vi "WLAN_Scrambler.vi"(11 "input bit stream":i8[](array[numeric])) -> (2 "scrambled bits":i8[](array[numeric]), 3 "scrambler initial bit":i8[](array[numeric]))   [LabVIEW 2022 SP3]
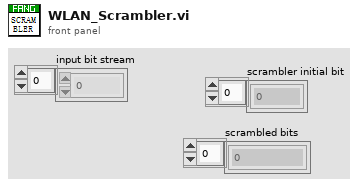
[diagram p1: front panel]
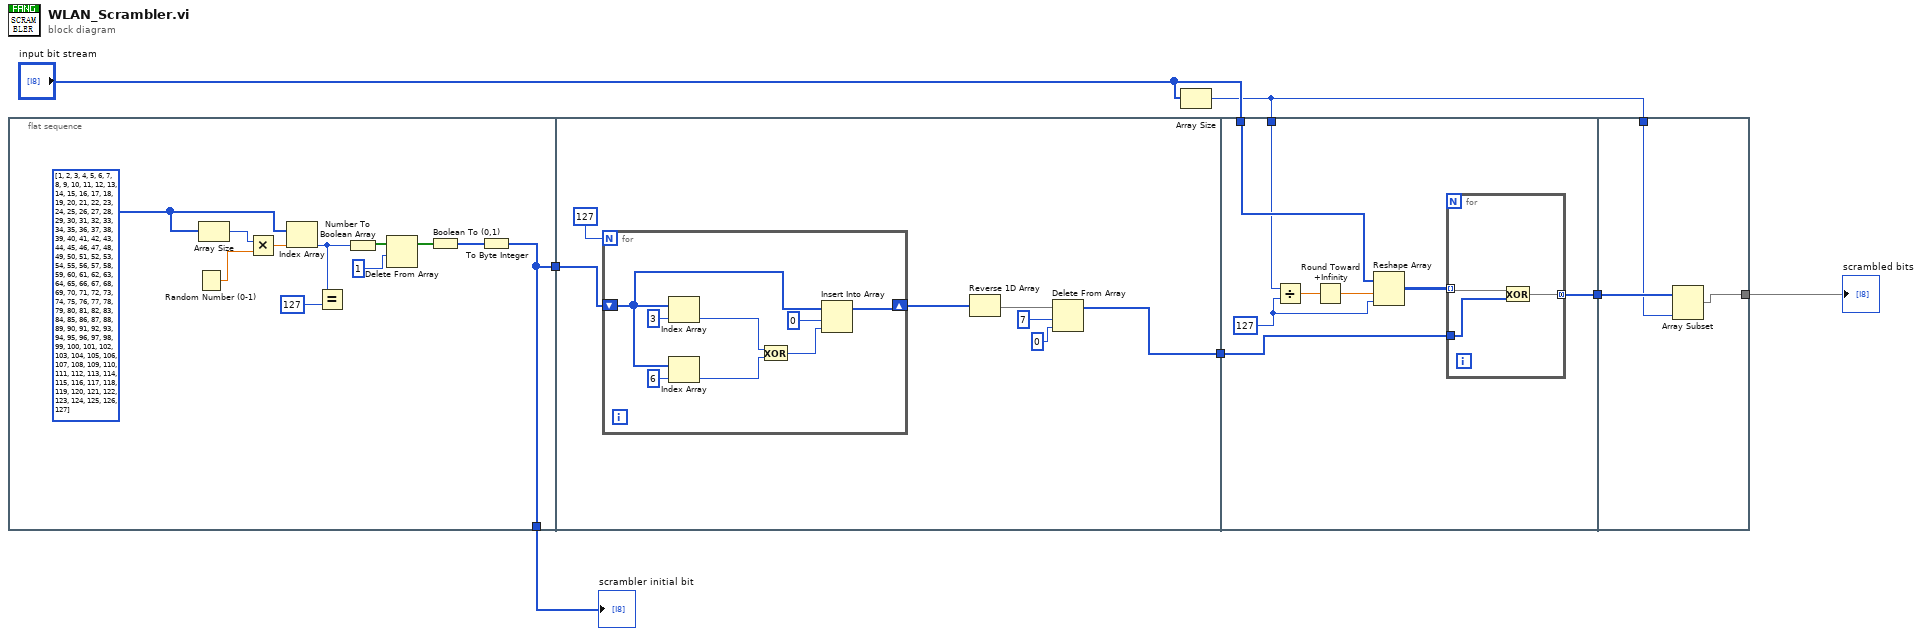
[diagram p0: block diagram]
diagram:
  n1 = flat-sequence {
    tunnel: [w8] -> w7
    tunnel: [w8] -> w6
    tunnel: w7 -> [w25]
    tunnel: [w19] -> w5
    tunnel: "input bit stream" -> [w40]
    tunnel: w5 -> [w36]
    tunnel: [w35] -> w3
    tunnel: w1 -> [w34]
    tunnel: [w45] -> w4
    tunnel: w3 -> [w47]
    tunnel: w1 -> [w46]
    frame #0 {
      w15 = i8[] [1, 2, 3, 4, 5, 6, 7, 8, 9, 10, 11, 12, 13, 14, 15, 16, 17, 18, 19, 20, 21, 22, 23, 24, 25, 26, 27, 28, 29, 30, 31, 32, 33, 34, 35, 36, 37, 38, 39, 40, 41, 42, 43, 44, 45, 46, 47, 48, 49, 50, 51, 52, 53, 54, 55, 56, 57, 58, 59, 60, 61, 62, 63, 64, 65, 66, 67, 68, 69, 70, 71, 72, 73, 74, 75, 76, 77, 78, 79, 80, 81, 82, 83, 84, 85, 86, 87, 88, 89, 90, 91, 92, 93, 94, 95, 96, 97, 98, 99, 100, 101, 102, 103, 104, 105, 106, 107, 108, 109, 110, 111, 112, 113, 114, 115, 116, 117, 118, 119, 120, 121, 122, 123, 124, 125, 126, 127] ("Array")
      n2 = Random Number (0-1)() -> (number: 0 to 1=w17:dbl)
      n3 = Array Size(array=w15) -> (size(s)=w18:i32)
      n4 = Multiply(x=w18, y=w17) -> (x*y=w16:dbl)
      n5 = Index Array(array=w15, index=w16) -> (element=w14:i8)
      n6 = Equal?(x=w14, y=i8 127) -> ()  [unwired: 1 out]
      n7 = Number To Boolean Array(number=w14) -> (Boolean array=w12:bool[])
      n8 = Delete From Array(array=w12, length=1) -> (array with subset deleted=w11:bool[])  [unwired: 1 in, 1 out]
      n9 = Boolean To (0,1)(Boolean=w11) -> (0, 1=w10:i16[])
      n10 = To Byte Integer(number=w10) -> (8bit integer=w8:i8[])
    }
    frame #1 {
      n11 = for {
        N: 127 -> [_]
        shift-right: [w26] -> w20
        shift-left: w25 -> [w29]
        n12 = Index Array(array=w29, index=3) -> (element=w31:i8)
        n13 = Index Array(array=w29, index=6) -> (element=w30:i8)
        n14 = Exclusive Or(1:w30, 2:w31) -> (0:w27:i8)
        n15 = Insert Into Array(array=w29, index=0, new element=w27) -> (w26:i8[])
      }
      n16 = Reverse 1D Array(array=w20) -> (reversed array=w21:i8[])
      n17 = Delete From Array(array=w21, length=7, index=0) -> (array with subset deleted=w19:i8[])  [unwired: 1 out]
    }
    frame #2 {
      w38 = 127
      n18 = Divide(x=w34, y=w38) -> (x/y=w41:dbl)
      n19 = Round Toward +Infinity(x=w41) -> (ceil(x): smallest int >= x=w39:dbl)
      n20 = Reshape Array(w40, w39, w38) -> (w37:i8[][])
      n21 = for {
        tunnel: w37 -> [w44] mode=indexing
        tunnel: w36 -> [w43]
        tunnel: [w42] -> w35 mode=concatenating
        n22 = Exclusive Or(1:w43, 2:w44) -> (0:w42:i8[])
      }
    }
    frame #3 {
      n23 = Array Subset(array=w47, length=w46) -> (w45:i8[])  [unwired: 1 in]
    }
  }
  n24 = Array Size(array="input bit stream") -> (size(s)=w1:i32)
  "scrambler initial bit" <- w6
  "scrambled bits" <- w4
